vi "CMD_ABS.vi"(6 "Gantry in":refnum<class "Gantry.lvclass">, 8 "error in (no error)":errorcluster, 10 "Arguments":string[](array[string]), 11 "gScript Interpreter in":refnum<class "gScript Interpreter.lvclass">) -> (0 "error out":errorcluster, 3 "gScript Interpreter out":refnum<class "gScript Interpreter.lvclass">, 4 "Gantry out":refnum<class "Gantry.lvclass">)   [LabVIEW 2023, in "gScript Interpreter.lvclass"]
uses:
  gScript Interpreter.lvclass
  Shared Components/Gantry Class/Gantry.lvclass
  Type Definitions/Memory Cell.ctl
  Type Definitions/Memory Cell Type Enum.ctl
  Shared Components/Vec3d Class/Vec3d.lvclass
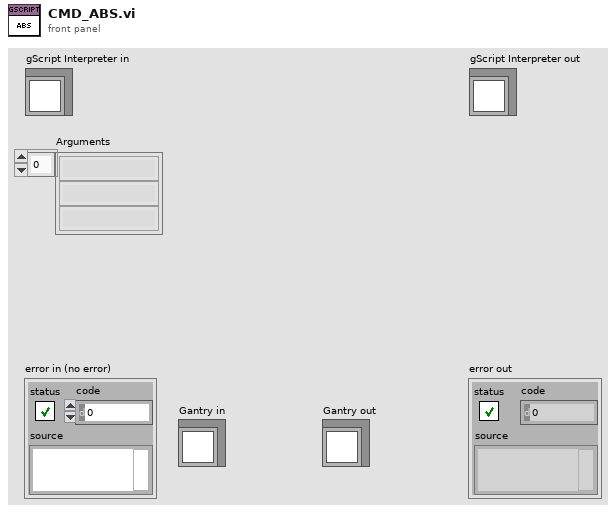
[diagram p1: front panel]
types:
  T1 = typedef "Memory Cell Type Enum.ctl" = enum16{"integer", "float", "vector", "rotation"}
  T2 = typedef "Memory Cell.ctl" = cluster{"type":T1, "x":dbl, "y":dbl, "z":dbl, "w":dbl}
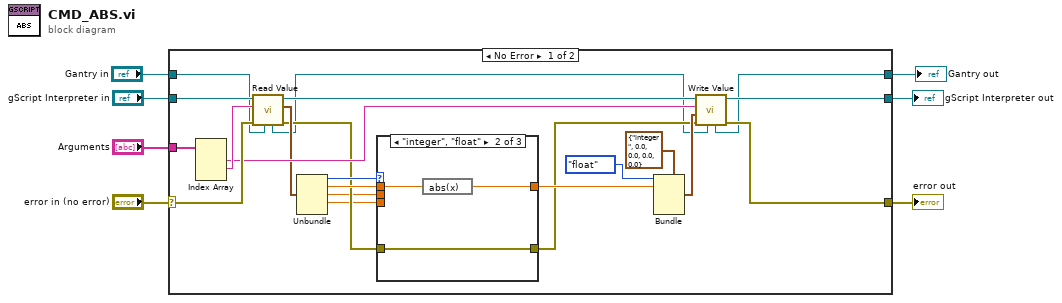
[diagram p0: block diagram]
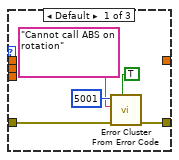
[diagram p2: hidden frame]
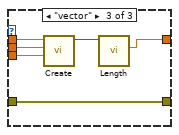
[diagram p3: hidden frame]
diagram:
  n1 = case shown="No Error" "error in (no error)" {
    selector: "error in (no error)" -> [w27 w46]
    tunnel: [w20 w46] -> w6
    tunnel: [w21 w45] -> w4
    tunnel: "gScript Interpreter in" -> [w28 w45]
    tunnel: "Arguments" -> [w29 _]
    tunnel: "Gantry in" -> [w10 w44]
    tunnel: [w8 w44] -> w1
    frame No Error {
      n2 = Index Array(array=w29) -> (element #1=w25:string, element #2=w26:string)  [unwired: 3 in, 1 out]
      n3 = call-dynamic "Read Value.vi"("Gantry in"=w10, "error in (no error)"=w27, "String in"=w26, "gScript Interpreter in"=w28) -> ("error out"=w14:errorcluster, "Memory Cell"=w24:T2, "gScript Interpreter out"=w19:refnum<class "gScript Interpreter.lvclass">, "Gantry out"=w9:refnum<class "Gantry.lvclass">)  [unwired: 4 in]
      n4 = Unbundle(w24) -> ("type"=w18:T1, "x"=w17:dbl, "y"=w12:dbl, "z"=w11:dbl)  [unwired: 1 out]
      n5 = case shown="\"integer\", \"float\"" w18 {
        tunnel: w17 -> [_ w37 w43]
        tunnel: [_ w36 w39] -> w16
        tunnel: w14 -> [w30 w35 w38]
        tunnel: [w34 w35 w38] -> w13
        tunnel: w12 -> [_ _ w42]
        tunnel: w11 -> [_ _ w41]
        frame Default {
          n6 = call <vilib>:"Error Cluster From Error Code.vi"("show call chain? (False)"=TRUE, "error in (no error)"=w30, "error message (\"\")"="Cannot call ABS on rotation" ("error message (\"\")"), "error code (0)"=5001) -> ("error out"=w34:errorcluster)  [unwired: 5 in]
        }
        frame "integer", "float" {
          n7 = expression code="abs(x)"(w37) -> (w36:dbl)
        }
        frame "vector" {
          n8 = call "Create.vi"("Z"=w41, "Y"=w42, "X"=w43) -> ("Vec3d Class out"=w40:refnum<class "Vec3d.lvclass">)  [unwired: 7 in, 1 out]
          n9 = call-dynamic "Length.vi"("Vec3d in"=w40) -> ("Length"=w39:dbl)  [unwired: 8 in, 2 out]
        }
      }
      n10 = Bundle(cluster=T2 {"type"=enum."integer", "x"=0.0, "y"=0.0, "z"=0.0, "w"=0.0} ("Memory Cell"), "type"=Memory_Cell_Type_Enum."float", "x"=w16) -> (w22:T2)  [unwired: 3 in]
      n11 = call-dynamic "Write Value.vi"("Gantry in"=w9, "error in (no error)"=w13, "Value"=w22, "Address"=w25, "gScript Interpreter in"=w19) -> ("error out"=w20:errorcluster, "gScript Interpreter out"=w21:refnum<class "gScript Interpreter.lvclass">, "Gantry out"=w8:refnum<class "Gantry.lvclass">)  [unwired: 4 in]
    }
    frame Error {
    }
  }
  "error out" <- w6
  "gScript Interpreter out" <- w4
  "Gantry out" <- w1
